vi "Log File.vi"(0 "File Path":path, 2 "Actions":T1, 7 "Message":string, 11 "Time Stamp?":bool=TRUE) -> ()   [LabVIEW 2020]
uses:
  Log File Type Defs/Log File Actions.ctl
panel:
  out "Error":errorcluster
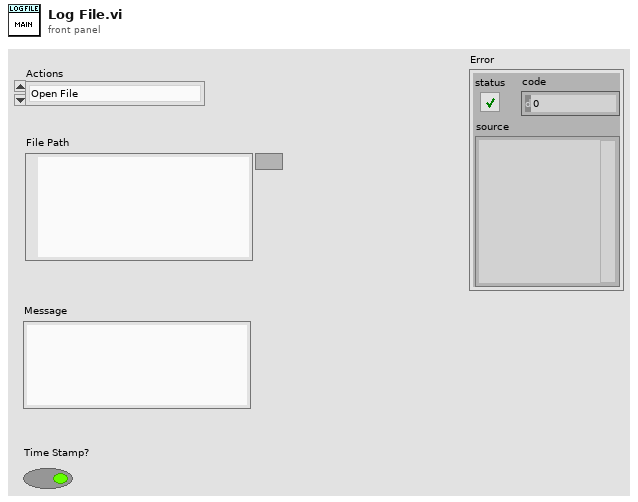
[diagram p1: front panel]
types:
  T1 = typedef "Log File Actions.ctl" = enum16{"Open File", "Write"}
  T2 = enum16{"open", "replace", "create", "open or create", "replace or create", "replace or create with confirmation"}
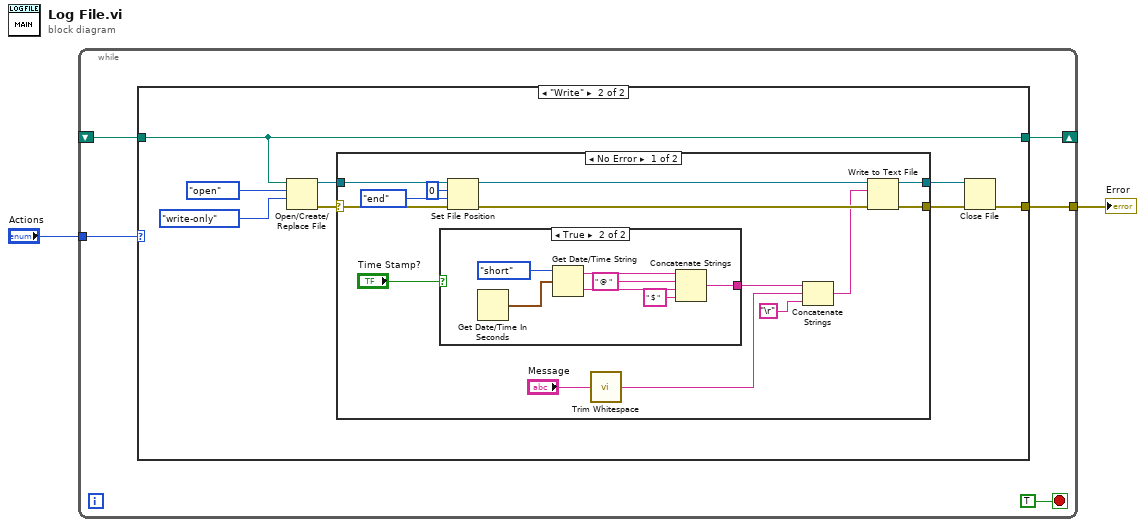
[diagram p0: block diagram]
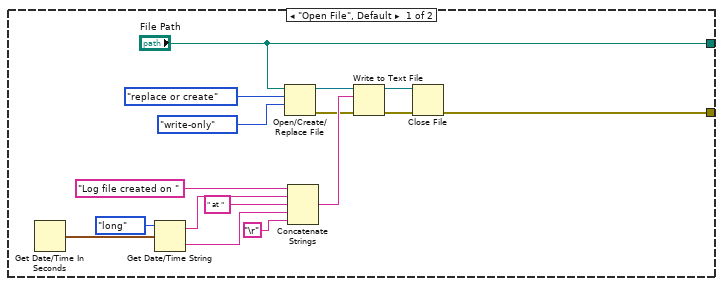
[diagram p2: hidden frame]
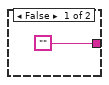
[diagram p3: hidden frame]
diagram:
  n1 = while {
    tunnel: "Actions" -> [w7]
    tunnel: [w5] -> w1
    shift-right: [w4] -> _
    shift-left: _ -> [w3]
    stop <- TRUE stop-if-true
    n2 = case shown="\"Write\"" w7 {
      tunnel: [w9 w25] -> w5
      tunnel: ["File Path" w24] -> w4
      tunnel: w3 -> [_ w24]
      frame "Open File", Default {
        n3 = Get Date/Time In Seconds() -> (seconds since 1Jan1904=w15:timestamp)
        n4 = Get Date/Time String(date format (0)=enum16{"short", "long", "abbreviated"}."long", seconds (now)=w15) -> (date string=w18:string, time string=w20:string)  [unwired: 1 in]
        n5 = Open/Create/Replace File(file path (use dialog)="File Path", operation (0:open)=T2."replace or create", access (0:read/write)=enum16{"read/write", "read-only", "write-only"}."write-only") -> (refnum out=w14:refnum<file>, error out=w12:errorcluster)  [unwired: 3 in, 1 out]
        n6 = Concatenate Strings("Log file created on ", w18, " at " ("string"), w20, "\r") -> (w13:string)
        n7 = Write to Text File(file (use dialog)=w14, text=w13, error in=w12) -> (refnum out=w11:refnum<file>, error out=w10:errorcluster)  [unwired: 1 in, 1 out]
        n8 = Close File(refnum=w11, error in=w10) -> (error out=w9:errorcluster)  [unwired: 1 out]
      }
      frame "Write" {
        n9 = Open/Create/Replace File(file path (use dialog)=w24, operation (0:open)=T2."open", access (0:read/write)=enum16{"read/write", "read-only", "write-only"}."write-only") -> (refnum out=w29:refnum<file>, error out=w28:errorcluster)  [unwired: 3 in, 1 out]
        n10 = case shown="No Error" w28 {
          selector: w28 -> [w39 w55]
          tunnel: w29 -> [w40 w54]
          tunnel: [w35 w55] -> w26
          tunnel: [w36 w54] -> w27
          frame No Error {
            n11 = case shown="True" "Time Stamp?" {
              tunnel: ["" w47] -> w43
              frame False {
              }
              frame True {
                n12 = Get Date/Time In Seconds() -> (seconds since 1Jan1904=w49:timestamp)
                n13 = Get Date/Time String(date format (0)=enum16{"short", "long", "abbreviated"}."short", seconds (now)=w49) -> (date string=w51:string, time string=w53:string)  [unwired: 1 in]
                n14 = Concatenate Strings(w51, " @ " ("string"), w53, " $ " ("string")) -> (w47:string)
              }
            }
            n15 = Set File Position(offset (in bytes) (0)=i64 0, refnum=w40, from (0:start)=enum16{"start", "end", "current"}."end", error in=w39) -> (refnum out=w38:refnum<file>, error out=w37:errorcluster)
            n16 = call <vilib>:"Trim Whitespace.vi"("string"="Message") -> ("trimmed string"=w42:string)  [unwired: 1 in]
            n17 = Concatenate Strings(w43, w42, "\r") -> (w34:string)
            n18 = Write to Text File(file (use dialog)=w38, text=w34, error in=w37) -> (refnum out=w36:refnum<file>, error out=w35:errorcluster)  [unwired: 1 in, 1 out]
          }
          frame Error {
          }
        }
        n19 = Close File(refnum=w27, error in=w26) -> (error out=w25:errorcluster)  [unwired: 1 out]
      }
    }
  }
  "Error" <- w1
